vi "ReferenceData.vi"(7 "Results":T2[](array[typedef]) {"Mesh_std" format="%#_13g"; "Mesh_mean" format="%#_13g"; "Order power spectra"."order 0" format="%.2p"; "Order power spectra"."delta order" format="%.2p"; "Order power spectra"."magnitude" format="%.2f"; "Power Spectrum / PSD"."magnitude" format="%.2p"; "Power Spectrum / PSD"."f0" format="%.2p"; "Power Spectrum / PSD"."df" format="%.2p"}, 8 "error in (no error)":errorcluster, 10 "DatatoRef in":T1) -> (0 "error out":errorcluster, 2 "DatatoRef out":T1)   [LabVIEW 2021]
uses:
  Typedefs/Results.ctl
  Typedefs/Detected peaks.ctl
  Typedefs/DataToRef.ctl
panel:
  in  "Init?":bool=TRUE
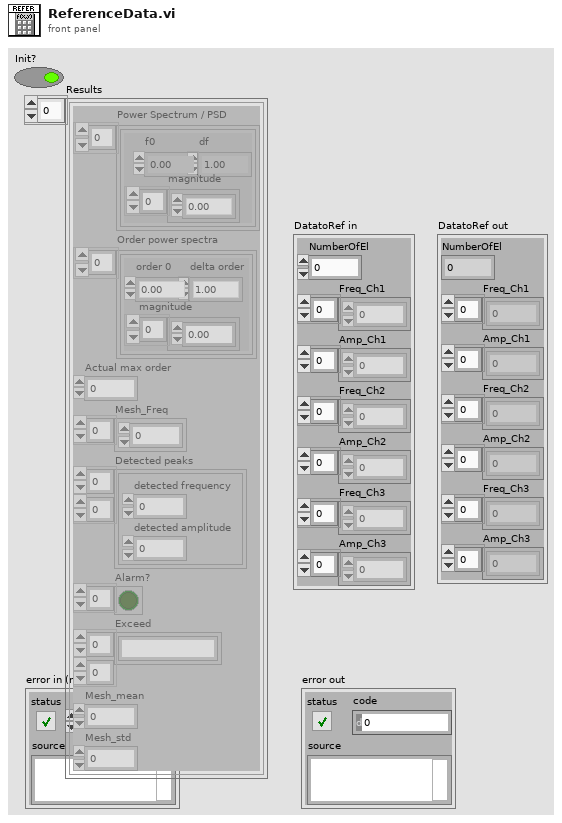
[diagram p1: front panel]
types:
  T1 = typedef "DataToRef.ctl" = cluster{"NumberOfEl":dbl, "Freq_Ch1":dbl[], "Amp_Ch1":dbl[], "Freq_Ch2":dbl[], "Amp_Ch2":dbl[], "Freq_Ch3":dbl[], "Amp_Ch3":dbl[]}
  T2 = typedef "Results.ctl" = cluster{"Power Spectrum / PSD":cluster{"f0":dbl, "df":dbl, "magnitude":dbl[]}[], "Order power spectra":cluster{"order 0":dbl, "delta order":dbl, "magnitude":dbl[]}[], "Actual max order":dbl, "Mesh_Freq":dbl[], "Detected peaks":T3[][], "Alarm?":bool[], "Exceed":string[][], "Mesh_mean":dbl, "Mesh_std":dbl}
  T3 = typedef "Detected peaks.ctl" = cluster{"detected frequency":dbl, "detected amplitude":dbl}
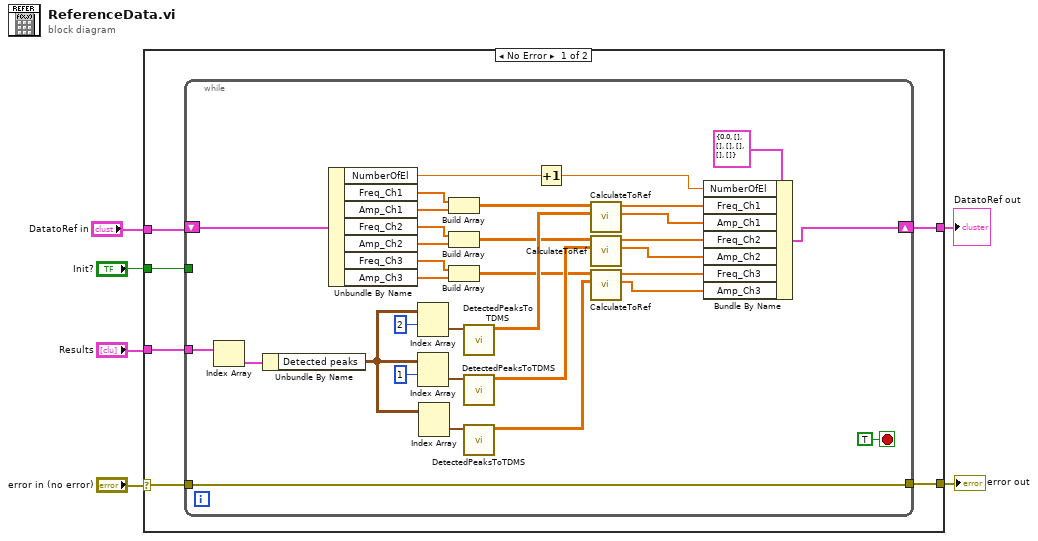
[diagram p0: block diagram]
diagram:
  n1 = case shown="No Error" "error in (no error)" {
    selector: "error in (no error)" -> [w11 w47]
    tunnel: [w10 w47] -> w5
    tunnel: "Results" -> [w12 _]
    tunnel: "Init?" -> [w9 _]
    tunnel: [w8 w46] -> w2
    tunnel: "DatatoRef in" -> [w7 w46]
    frame No Error {
      n2 = while {
        shift-right: [w43] -> w8
        shift-left: w7 -> [w40]
        tunnel: w12 -> [w42]
        tunnel: [w41] -> w10
        tunnel: w11 -> [w41]
        tunnel: w9 -> [_]
        stop <- TRUE stop-if-true
        n3 = Index Array(array=w42) -> (element=w30:T2)  [unwired: 1 in]
        n4 = Unbundle By Name(w30) -> ("Detected peaks"=w31:T3[][])
        n5 = Unbundle By Name(w40) -> ("NumberOfEl"=w13:dbl, "Freq_Ch1"=w23:dbl[], "Amp_Ch1"=w22:dbl[], "Freq_Ch2"=w20:dbl[], "Amp_Ch2"=w19:dbl[], "Freq_Ch3"=w17:dbl[], "Amp_Ch3"=w16:dbl[])
        n6 = Index Array(array=w31, index (row)=2) -> (element=w36:T3[])  [unwired: 1 in]
        n7 = Index Array(array=w31, index (row)=1) -> (element=w35:T3[])  [unwired: 1 in]
        n8 = Index Array(array=w31) -> (element=w33:T3[])  [unwired: 2 in]
        n9 = Build Array(w23, w22) -> (w21:dbl[][])
        n10 = Build Array(w20, w19) -> (w18:dbl[][])
        n11 = Build Array(w17, w16) -> (w15:dbl[][])
        n12 = call "DetectedPeaksToTDMS.vi"("Detected peaks"=w36) -> ("Array"=w29:dbl[][])  [unwired: 10 in]
        n13 = call "DetectedPeaksToTDMS.vi"("Detected peaks"=w35) -> ("Array"=w28:dbl[][])  [unwired: 10 in]
        n14 = call "DetectedPeaksToTDMS.vi"("Detected peaks"=w33) -> ("Array"=w14:dbl[][])  [unwired: 10 in]
        n15 = Increment(x=w13) -> (x+1=w44:dbl)
        n16 = call "CalculateToRef.vi"("New Data"=w29, "Old Data"=w21) -> ("Amlitude"=w37:dbl[], "Frequency"=w38:dbl[])  [unwired: 8 in]
        n17 = call "CalculateToRef.vi"("New Data"=w28, "Old Data"=w18) -> ("Amlitude"=w26:dbl[], "Frequency"=w27:dbl[])  [unwired: 8 in]
        n18 = call "CalculateToRef.vi"("New Data"=w14, "Old Data"=w15) -> ("Amlitude"=w24:dbl[], "Frequency"=w25:dbl[])  [unwired: 8 in]
        n19 = Bundle By Name(cluster=T1 {"NumberOfEl"=0.0, "Freq_Ch1"=[], "Amp_Ch1"=[], "Freq_Ch2"=[], "Amp_Ch2"=[], "Freq_Ch3"=[], "Amp_Ch3"=[]}, "NumberOfEl"=w44, "Freq_Ch1"=w38, "Amp_Ch1"=w37, "Freq_Ch2"=w27, "Amp_Ch2"=w26, "Freq_Ch3"=w25, "Amp_Ch3"=w24) -> (w43:T1)
      }
    }
    frame Error {
    }
  }
  "error out" <- w5
  "DatatoRef out" <- w2
